vi "Read TKEEP Core.vi"(11 "niInstr AXI4-Stream Reader FXP64x2 v1 FPGA in":refnum<class "niInstr AXI4-Stream Reader FXP64x2 v1 FPGA.lvclass">) -> (2 "value":bool[](array[boolean]), 3 "niInstr AXI4-Stream Reader FXP64x2 v1 FPGA out":refnum<class "niInstr AXI4-Stream Reader FXP64x2 v1 FPGA.lvclass">)   [LabVIEW 2015, in "niInstr AXI4-Stream Reader FXP64x2 v1 FPGA.lvclass"]
doc: "<B>Input Parameters</B>\n\n<B>niInstr AXI4-Stream Reader FXP64x2 v1 FPGA in</B> takes in a reference to the AXI4-Stream Reader from the previous VI."
uses:
  <instrlib>/_niInstr/CLIP Adapters/v1/FPGA/AXI4-Stream/Reader FXP64x2/niInstr AXI4-Stream Reader FXP64x2 v1 FPGA.lvclass
  <instrlib>/_niInstr/CLIP Adapters/v1/FPGA/AXI4-Stream/Reader FXP64x2/niInstr AXI4-Stream Reader FXP64x2 v1 FPGA.lvclass/niInstr AXI4-Stream Reader FXP64x2 v1 FPGA.ctl
  <instrlib>/_niInstr/Data Formatting/v1/FPGA/Private/Convert/U16 array to Boolean Array.vi
  <vilib>/rvi/eio/common/nirviEmuTemplateMethod_errors.vi
  <vilib>/eio/EIONode/EIONode.xnode
  <instrlib>/_niInstr/Data Formatting/v1/FPGA/niInstr Data Formatting v1 FPGA.lvlib
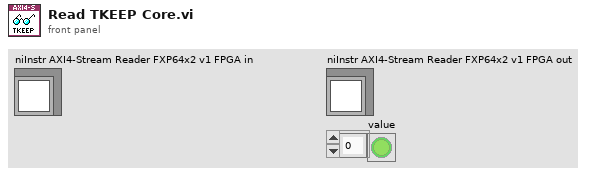
[diagram p1: front panel]
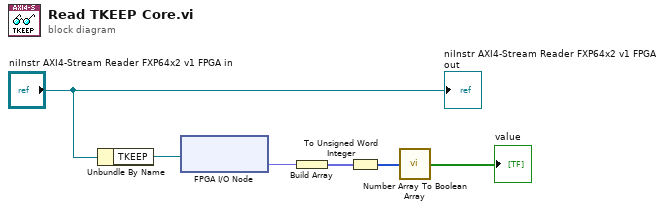
[diagram p0: block diagram]
diagram:
  n1 = Unbundle By Name("niInstr AXI4-Stream Reader FXP64x2 v1 FPGA in") -> ("TKEEP"=w5:refnum<k21>)
  n2 = xnode "FPGA I/O Node"("FPGA I/O In"=w5) -> ("I/O Item"=w4:fxp<+,16,16>)  [unwired: 1 out]
  n3 = Build Array(w4) -> (w3:fxp<+,16,16>[])
  n4 = To Unsigned Word Integer(number=w3) -> (unsigned 16bit integer=w2:u16[])
  n5 = call-poly <instrlib>:"Number Array To Boolean Array.vi"("data in"=w2) -> ("data out"=→"value":bool[])  [unwired: 14 in]
  "niInstr AXI4-Stream Reader FXP64x2 v1 FPGA out" <- "niInstr AXI4-Stream Reader FXP64x2 v1 FPGA in"
